vi "Substract.vi"(8 "error in (no error)":errorcluster, 11 "UPNCalculator in":refnum<class "UPNCalculator.lvclass">) -> (0 "error out":errorcluster, 3 "UPNCalculator out":refnum<class "UPNCalculator.lvclass">)   [LabVIEW 2012, in "UPNCalculator Actor.lvlib" / "UPNCalculator.lvclass"]
doc: "Poo 2 elements from stack, add them and put result back to stack."
uses:
  UPNCalculator.lvclass
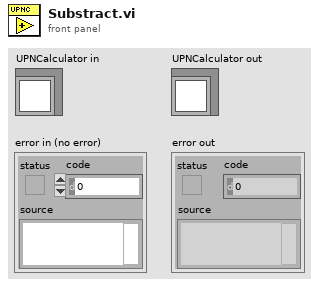
[diagram p1: front panel]
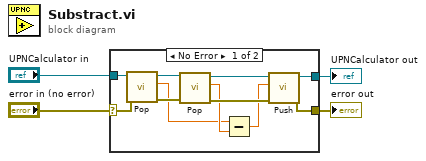
[diagram p0: block diagram]
diagram:
  n1 = case shown="No Error" "error in (no error)" {
    selector: "error in (no error)" -> [w6 w17]
    tunnel: [w5 w17] -> w3
    tunnel: [w12 w16] -> w1
    tunnel: "UPNCalculator in" -> [w13 w16]
    frame No Error {
      n2 = call "Pop.vi"("error in (no error)"=w6, "UPNCalculator in"=w13) -> ("error out"=w11:errorcluster, "Element"=w8:dbl, "UPNCalculator out"=w15:refnum<class "UPNCalculator.lvclass">)  [unwired: 7 in]
      n3 = call "Pop.vi"("error in (no error)"=w11, "UPNCalculator in"=w15) -> ("error out"=w10:errorcluster, "Element"=w9:dbl, "UPNCalculator out"=w14:refnum<class "UPNCalculator.lvclass">)  [unwired: 7 in]
      n4 = Subtract(x=w8, y=w9) -> (x-y=w7:dbl)
      n5 = call "Push.vi"("error in (no error)"=w10, "Element"=w7, "UPNCalculator in"=w14) -> ("error out"=w5:errorcluster, "UPNCalculator out"=w12:refnum<class "UPNCalculator.lvclass">)  [unwired: 7 in]
    }
    frame Error {
    }
  }
  "error out" <- w3
  "UPNCalculator out" <- w1
